vi "readTPDO.vi"(0 "OrionBMS.lvclass":refnum<class "OrionBMSClass.lvclass">, 2 "TPDO object in":refnum<k20>, 3 "error in (no error)":errorcluster) -> (5 "new data?":bool, 7 "OrionBMS.lvclass":refnum<class "OrionBMSClass.lvclass">, 8 "TPDO data":u8[](array[numeric]), 9 "TPDO object out":refnum<k20>, 10 "error out":errorcluster)   [LabVIEW 2018, in "OrionBMSClass.lvclass"]
uses:
  OrionBMSClass.lvclass
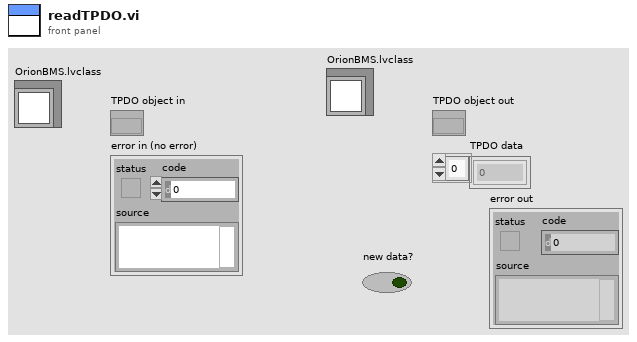
[diagram p1: front panel]
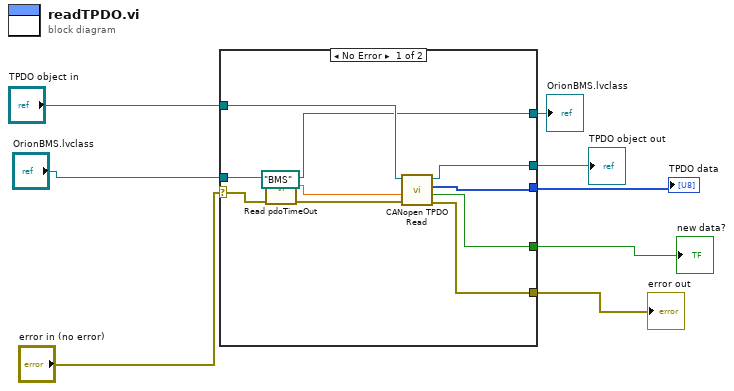
[diagram p0: block diagram]
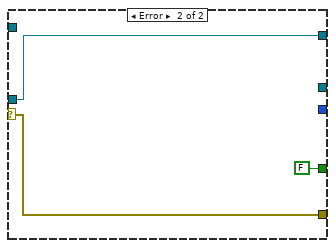
[diagram p2: hidden frame]
diagram:
  n1 = case shown="No Error" "error in (no error)" {
    selector: "error in (no error)" -> [w17 w19]
    tunnel: "OrionBMS.lvclass" -> [w18 w21]
    tunnel: "TPDO object in" -> [w16 _]
    tunnel: [w13 w21] -> w5
    tunnel: [w12 _] -> w4
    tunnel: [w11 _] -> w3
    tunnel: [w10 FALSE ("new data?")] -> w1
    tunnel: [w9 w19] -> w2
    frame No Error {
      (unwired) path "BMS"
      n2 = call-dynamic "Read pdoTimeOut.vi"("error in (no error)"=w17, "OrionBMS in"=w18) -> ("error out"=w14:errorcluster, "pdoTimeOut"=w15:dbl, "OrionBMS out"=w13:refnum<class "OrionBMSClass.lvclass">)  [unwired: 7 in]
      n3 = call <vilib>:"CANopen TPDO Read.vi"("error in (no error)"=w14, "timeout (0s)"=w15, "TPDO object in"=w16) -> ("error out"=w9:errorcluster, "new data?"=w10:bool, "data"=w11:u8[], "TPDO object out"=w12:refnum<k20>)  [unwired: 4 in, 1 out]
    }
    frame Error {
    }
  }
  "OrionBMS.lvclass" <- w5
  "TPDO object out" <- w4
  "TPDO data" <- w3
  "error out" <- w2
  "new data?" <- w1
